vi "Q_MGR.vi"(0 "QSTATES":cluster{"Data":variant, "MainState":T1}[](array[cluster]), 2 "QRef":refnum<queue>, 11 "Error IN":errorcluster, 12 "FNs":enum16{"Back", "Front", "Replace"}(ring)) -> (15 "Error OUT":errorcluster)   [LabVIEW 2010]
uses:
  types/MainStates.ctl
  types/MainStateQueueType.ctl
  MainGlobalConstants.vi
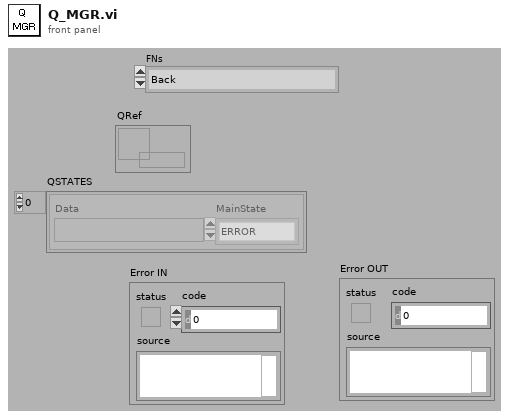
[diagram p1: front panel]
types:
  T1 = typedef "MainStates.ctl" = enum16{"initMain", "insertSubVI", "startSubVI", "stopSubVI", "Exit", "ERROR", "idle"}
  T2 = typedef "MainStateQueueType.ctl" = cluster{"Data":variant, "MainState":T1}
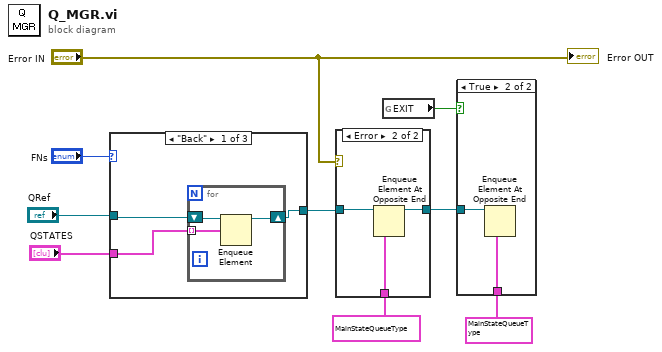
[diagram p0: block diagram]
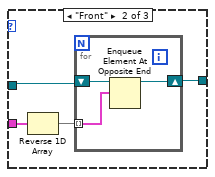
[diagram p4: hidden frame]
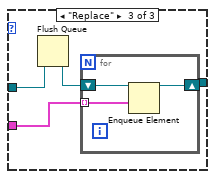
[diagram p5: hidden frame]
diagram:
  n1 = case shown="\"Back\"" "FNs" {
    tunnel: "QSTATES" -> [w11 w19 w24]
    tunnel: "QRef" -> [w10 w17 w26]
    tunnel: [w12 w16 w23] -> w8
    frame "Back" {
      n2 = for {
        shift-right: [w14] -> w12
        shift-left: w10 -> [w15]
        tunnel: w11 -> [w13] mode=indexing
        n3 = Enqueue Element(queue=w15, element=w13) -> (queue out=w14:refnum<queue>)  [unwired: 1 in, 3 out]
      }
    }
    frame "Front" {
      n4 = Reverse 1D Array(array=w19) -> (reversed array=w18:cluster{"Data":variant, "MainState":T1}[])
      n5 = for {
        tunnel: w18 -> [w21] mode=indexing
        shift-right: [w20] -> w16
        shift-left: w17 -> [w22]
        n6 = Enqueue Element At Opposite End(queue=w22, element=w21) -> (queue out=w20:refnum<queue>)  [unwired: 1 in, 3 out]
      }
    }
    frame "Replace" {
      n7 = Flush Queue(queue=w26) -> (queue out=w25:refnum<queue>)  [unwired: 1 in, 2 out]
      n8 = for {
        tunnel: w24 -> [w28] mode=indexing
        shift-right: [w27] -> w23
        shift-left: w25 -> [w29]
        n9 = Enqueue Element(queue=w29, element=w28) -> (queue out=w27:refnum<queue>)  [unwired: 2 in, 2 out]
      }
    }
  }
  n10 = case shown="Error" "Error IN" {
    tunnel: w8 -> [w30 w33]
    tunnel: [w30 w32] -> w7
    tunnel: T2 {"Data"=variant, "MainState"=enum."ERROR"} ("MainStateQueue") -> [_ w31]
    frame No Error {
    }
    frame Error {
      n11 = Enqueue Element At Opposite End(queue=w33, element=w31) -> (queue out=w32:refnum<queue>)  [unwired: 1 in, 3 out]
    }
  }
  n12 = global read "MainGlobalConstants.vi" "EXIT"() -> (w5:bool)
  n13 = case shown="True" w5 {
    tunnel: w7 -> [_ w35]
    tunnel: T2 {"Data"=variant, "MainState"=enum."Exit"} ("MainStateQueue") -> [_ w34]
    frame False {
    }
    frame True {
      n14 = Enqueue Element At Opposite End(queue=w35, element=w34) -> ()  [unwired: 1 in, 4 out]
    }
  }
  "Error OUT" <- "Error IN"
